vi "SFP_SwitchACIR.vi"(8 "error in (no error)":errorcluster, 11 "ACIR Instrument":refnum<class "ACIR Instrument.lvclass">) -> ()   [LabVIEW 2025, in "ACIR.lvlib" / "ACIR Instrument.lvclass"]
doc: "Copyright 2017 National Instruments Corporation\n\nLicensed under the Apache License, Version 2.0 (the \"License\"); you may not use this file except in compliance with the License. You may obtain a copy of the License at http://www.apache.org/licenses/LICENSE-2.0\nUnless required by applicable law or agreed to in writing, software distributed under the License is distributed on an \"AS IS\" BASIS, WITHOUT WARRANTIES OR CONDITIONS OF ANY KIND, either express or implied. See the License for the specific language governing permissions and limitations under the License."
uses:
  ACIR Instrument.lvclass
  ACIR Instrument.lvclass/ACIR Instrument.ctl
  ACIR configuration/ACIR configuration.lvclass
panel:
  out "Channels":T1(array[cluster]) {"Measurement" format="%#_4p"}
  out "Instrument":string caption="Instrument ::"
  # "ch"
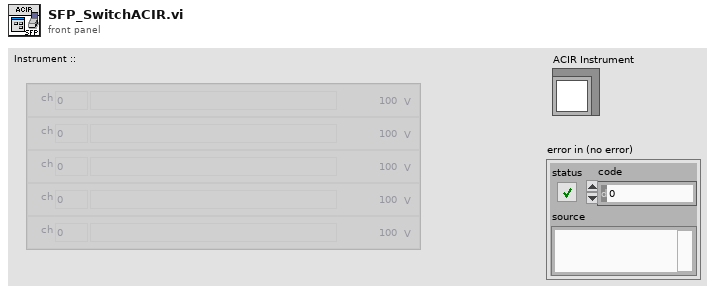
[diagram p1: front panel]
types:
  T1 = cluster{"Channel Alias":string, "Index":i32, "Measurement":dbl}[]
  T2 = enum32{"Invalid", "Default", "Floating", "Floating/Auto-Hide", "Modal"}
  T3 = typedef "Abstract Engine.lvlibp/Instrument configuration.lvclass/Default Instrument.ctl" = cluster{"Type":string, "Address":string, "SW Alias":string, "Description":string, "Enabled":bool}
  T4 = cluster{"Channel Alias":string, "Index":i32, "Measurement":dbl}
  T5 = typedef "Abstract Engine.lvlibp/Abstract Instrument.lvclass/Channel.ctl" = cluster{"Alias":string, "DataType":enum16{"Anaolg Input", "Waveform"}, "Unit":enum16{"---", "V", "A", "Ohm", "Hz", "uF", "degC", "deg"}, "Upper limit":dbl, "Lower limit":dbl, "Measurement":variant}
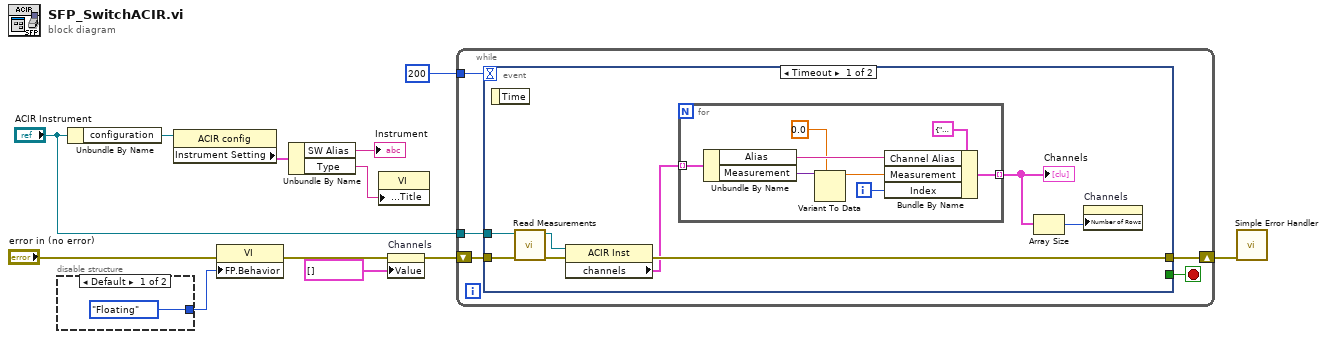
[diagram p0: block diagram]
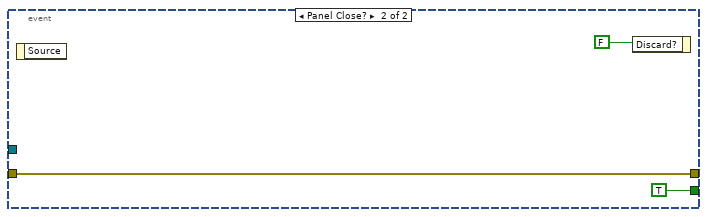
[diagram p2: hidden frame]
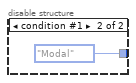
[diagram p3: hidden frame]
diagram:
  n1 = disable-structure shown="Default" {
    disable-tunnel: [T2."Floating" ("Front Panel Window:Behavior") T2."Modal" ("Front Panel Window:Behavior")] -> w10
    frame condition #0 (active) {
    }
    frame condition #1 {
    }
  }
  n2 = Unbundle By Name("ACIR Instrument") -> ("configuration"=w8:refnum<class "ACIR configuration.lvclass">)
  n3 = property class="ACIR config"(reference=w8) -> ("Instrument Setting"=w7:T3)  [unwired: 1 in, 2 out]
  n4 = property class="VI"(error in="error in (no error)", "FP.Behavior"=w10) -> (error out=w3:errorcluster)  [unwired: 1 in, 1 out]
  n5 = Unbundle By Name(w7) -> ("SW Alias"=→"Instrument":string, "Type"=w11:string)
  n6 = property class="VI"("Front Panel.Title"=w11) -> ()  [unwired: 2 in, 2 out]
  n7 = property on="Channels" class="Arr (strict)"(error in=w3, "Value"=T1 [] ("Channels")) -> (error out=w2:errorcluster)  [unwired: 1 in, 1 out]
  n8 = while {
    shift-right: [w17] -> w1
    shift-left: w2 -> [w18]
    tunnel: 200 -> [w15]
    tunnel: "ACIR Instrument" -> [w16]
    stop <- w19 stop-if-true
    n9 = event shown="[0] Timeout" {
      selector: _ -> [_ _]
      dyn-events: _ -> [_ _]
      timeout: w15 -> [_ _]
      tunnel: [_ TRUE] -> w19
      tunnel: [w22 w36] -> w17
      tunnel: w18 -> [w26 w36]
      tunnel: w16 -> [w23 _]
      event Timeout {
        n10 = event-data() -> ()  [unwired: 1 in, 1 out]
        n11 = call-dynamic "Read Measurements.vi"("error in (no error)"=w26, "ACIR Instrument in"=w23) -> ("error out"=w25:errorcluster, "ACIR Instrument out"=w21:refnum<class "ACIR Instrument.lvclass">)  [unwired: 7 in, 1 out]
        n12 = property class="ACIR Inst"(reference=w21, error in=w25) -> (error out=w22:errorcluster, "channels"=w20:T5[])  [unwired: 1 out]
        n13 = for {
          tunnel: [w35] -> w24 mode=indexing
          tunnel: w20 -> [w32] mode=indexing
          i -> [w34]
          n14 = Unbundle By Name(w32) -> ("Alias"=w31:string, "Measurement"=w30:variant)
          n15 = Variant To Data(type=0.0 ("Measurement"), Variant=w30) -> (data=w28:dbl)  [unwired: 1 in, 1 out]
          n16 = Bundle By Name(cluster=T4 {"Channel Alias"="", "Index"=0, "Measurement"=0.0} ("Channel"), "Channel Alias"=w31, "Measurement"=w28, "Index"=w34) -> (w35:T4)
        }
        "Channels" <- w24
        n17 = Array Size(array=w24) -> (size(s)=w27:i32)
        n18 = property on="Channels" class="Arr (strict)"("Number of Rows"=w27) -> ()  [unwired: 2 in, 2 out]
      }
      event Panel Close? {
        n19 = event-data() -> ()  [unwired: 1 in, 1 out]
        n20 = event-data("Discard?"=FALSE) -> ()  [unwired: 1 in, 1 out]
      }
    }
  }
  n21 = call <vilib>:"Simple Error Handler.vi"("error in (no error)"=w1) -> ()  [unwired: 4 in, 5 out]
